vi "Tracepoint_CreateDataEvent.vi"(8 "error in (no error)":errorcluster, 9 "data":T4, 10 "data event config":T1, 11 "Qbus":refnum<class "Qbus.lvclass">) -> (0 "error out":errorcluster)   [LabVIEW 2017, in "EmsaDataEventCreator.lvlib"]
uses:
  <vilib>/addons/InsightCM/Devices/Shared/Emsa/EmsaDataEventCreator/EmsaDataEventCreator.lvlib
  <vilib>/addons/Qbus/Qbus.lvclass
  <vilib>/addons/InsightCM/Devices/Shared/Common/DataFlow/controls/Data.ctl
  <vilib>/addons/InsightCM/Utilities/DataAccessors/controls/wfmSGL_DVR.ctl
  <vilib>/addons/PointValueMap/controls/PointMap.ctl
  <vilib>/addons/InsightCM/Devices/Shared/Common/DataFlow/controls/Type.ctl
  <vilib>/addons/InsightCM/Devices/Shared/Emsa/EmsaDataEventCreator/controls/DataEventConfig.ctl
  <vilib>/addons/InsightCM/Devices/Shared/Emsa/EmsaDataEventCreator/controls/SweepParams.ctl
  <vilib>/addons/TraceLogger/TraceLogger.lvlib
  <vilib>/addons/PointValueMap/PointValueMap.lvlib
  <vilib>/addons/InsightCM/Devices/Shared/Common/DataFlow/DataFlow.lvlib
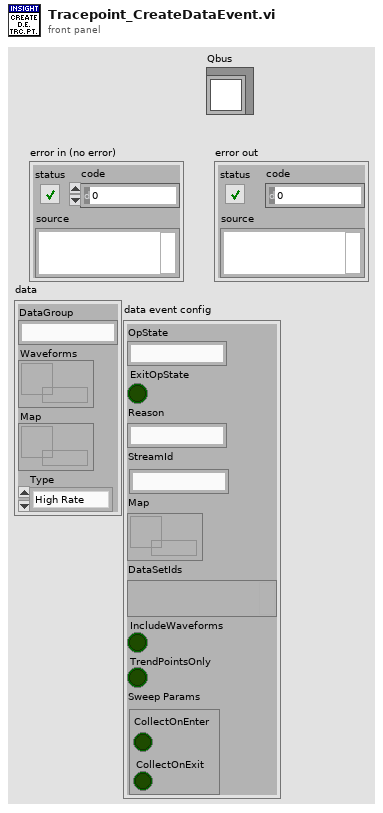
[diagram p1: front panel]
types:
  T1 = typedef "EmsaDataEventCreator.lvlib/DataEventConfig.ctl" = cluster{"OpState":string, "ExitOpState":bool, "Reason":string, "StreamId":string, "Map":T2, "DataSetIds":variant, "IncludeWaveforms":bool, "TrendPointsOnly":bool, "Sweep Params":T3}
  T2 = typedef "PointValueMap.lvlib/PointMap.ctl" = refnum<data-value>
  T3 = typedef "EmsaDataEventCreator.lvlib/SweepParams.ctl" = cluster{"CollectOnEnter":bool, "CollectOnExit":bool}
  T4 = typedef "DataFlow.lvlib/Data.ctl" = cluster{"DataGroup":string, "Waveforms":T5, "Map":T2, "Type":T6}
  T5 = typedef "wfmSGL_DVR.ctl" = refnum<data-value>
  T6 = typedef "DataFlow.lvlib/Type.ctl" = enum16{"High Rate", "Low Rate", "Burst Mode"}
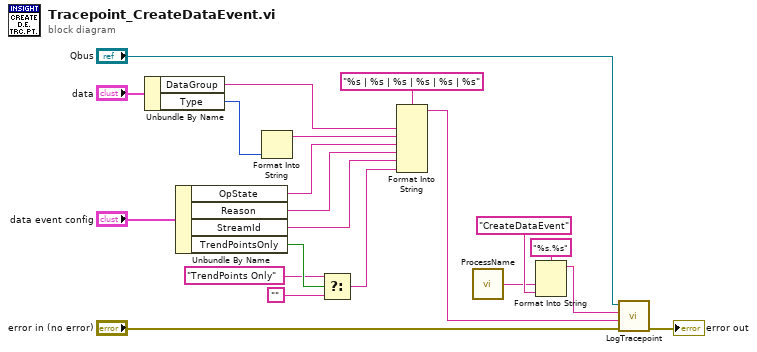
[diagram p0: block diagram]
diagram:
  n1 = Unbundle By Name("data") -> ("DataGroup"=w5:string, "Type"=w2:T6)
  n2 = Unbundle By Name("data event config") -> ("OpState"=w7:string, "Reason"=w15:string, "StreamId"=w12:string, "TrendPointsOnly"=w11:bool)
  n3 = Format Into String(w2) -> (resulting string=w1:string)  [unwired: 3 in, 1 out]
  n4 = Select(t="TrendPoints Only" ("StreamId"), s=w11, f="") -> (s? t:f=w9:string)
  n5 = Format Into String(format string="%s | %s | %s | %s | %s | %s", w5, w1, w7, w15, w12, w9) -> (resulting string=w14:string)  [unwired: 2 in, 1 out]
  n6 = call <vilib>:"ProcessName.vi"() -> ("process name"=w3:string)  [unwired: 5 in]
  n7 = Format Into String(format string="%s.%s", w3, "CreateDataEvent" ("tracepoint")) -> (resulting string=w17:string)  [unwired: 2 in, 1 out]
  n8 = call <vilib>:"LogTracepoint.vi"("error in (no error)"="error in (no error)", "log string"=w14, "tracepoint"=w17, "qbus in"="Qbus") -> ("error out"=→"error out":errorcluster)  [unwired: 6 in, 1 out]
